vi "demo subvi fileio.vi"(8 "exception in":T1 {"code" format="%.0x"}, 11 "file path":path=path "test.txt") -> (0 "exception out":T1 {"code" format="%.0x"}, 3 "text":string)   [LabVIEW 2013]
uses:
  errors/exception.ctl
  errors/context.ctl
  <vilib>/Utility/VariantDataType/GetTypeInfo.vi
  errors/Variant Repository/Write Variant Repository/Write Exception Property.xnode
  errors/error groups/files/file errors.lvlib
  errors/exception.lvlib
  <vilib>/Utility/VariantDataType/VariantType.lvlib
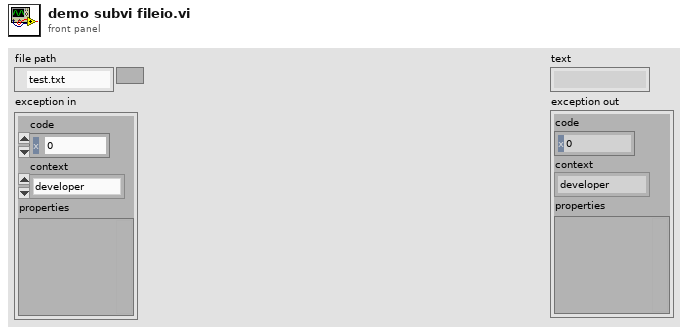
[diagram p1: front panel]
types:
  T1 = typedef "exception.lvlib/exception.ctl" = cluster{"code":i32, "context":T2, "properties":variant}
  T2 = typedef "exception.lvlib/context.ctl" = enum16{"developer", "user interface", "standard", "limited", "deterministic"}
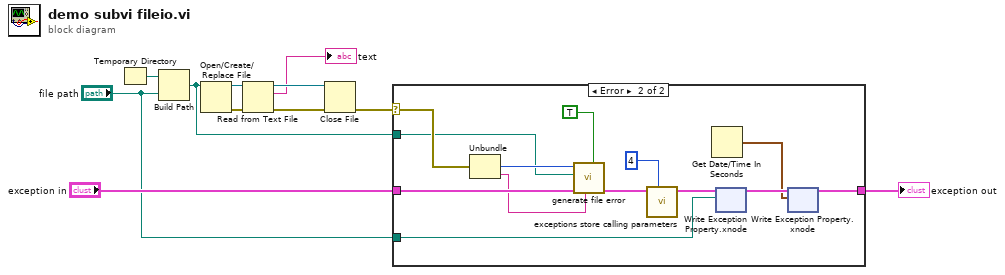
[diagram p0: block diagram]
diagram:
  n1 = Temporary Directory() -> (w11:path)
  n2 = Build Path(base path=w11, name or relative path="file path") -> (appended path=w3:path)
  n3 = Open/Create/Replace File(file path (use dialog)=w3) -> (refnum out=w10:refnum<file>, error out=w9:errorcluster)  [unwired: 5 in, 1 out]
  n4 = Read from Text File(file (use dialog)=w10, error in=w9) -> (refnum out=w8:refnum<file>, text=→"text":string, error out=w7:errorcluster)  [unwired: 2 in, 1 out]
  n5 = Close File(refnum=w8, error in=w7) -> (error out=w4:errorcluster)  [unwired: 1 out]
  n6 = case shown="Error" w4 {
    selector: w4 -> [_ w23]
    tunnel: "exception in" -> [w12 w25]
    tunnel: [w12 w14] -> w2
    tunnel: w3 -> [_ w20]
    tunnel: "file path" -> [_ w16]
    frame No Error {
    }
    frame Error {
      n7 = Unbundle(w23) -> ("code"=w22:i32, "source"=w21:string)  [unwired: 1 out]
      n8 = call "generate file error.vi"("call chain?"=TRUE, "source"=w21, "exception in"=w25, "file path"=w20, "file error"=w22) -> ("exception"=w19:T1)  [unwired: 6 in]
      n9 = call "exceptions store calling parameters.vi"("levels"=u8 4, "exception in"=w19) -> ("exception out"=w17:T1)  [unwired: 9 in]
      n10 = Get Date/Time In Seconds() -> (seconds since 1Jan1904=w13:timestamp)
      n11 = xnode "Write Exception Property.xnode"("exception in"=w17, "Value"=w16) -> ("exception out"=w15:T1)  [unwired: 1 in, 1 out]
      n12 = xnode "Write Exception Property.xnode"("exception in"=w15, "Value"=w13) -> ("exception out"=w14:T1)  [unwired: 1 in, 1 out]
    }
  }
  "exception out" <- w2
